vi "Camera Disconnect.vi"(8 "error in":errorcluster, 11 "Refnum in":T1) -> (0 "error out":errorcluster)   [LabVIEW 2015]
uses:
  <vilib>/userdefined/High Color/IMAQdx.ctl
  <vilib>/vision/driver/NI_Vision_Acquisition_Software.lvlib
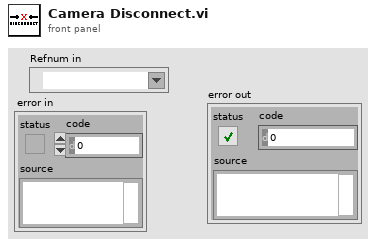
[diagram p1: front panel]
types:
  T1 = typedef "IMAQdx.ctl" = refnum<k21>
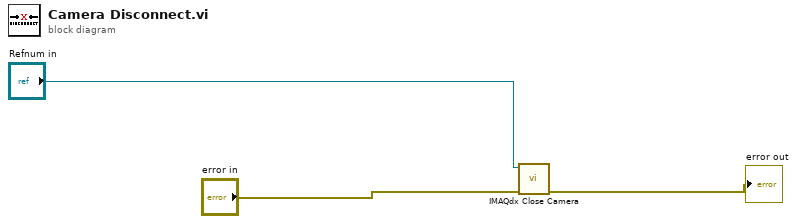
[diagram p0: block diagram]
diagram:
  n1 = call <vilib>:"IMAQdx Close Camera.vi"("error in"="error in", "Session In"="Refnum in") -> ("error out"=→"error out":errorcluster)  [unwired: 9 in]
